vi "Error Clusters and Error Handling.vi"() -> ()   [LabVIEW 2023]
uses:
  <vilib>/Utility/error.llb/DialogType.ctl
panel:
  out "source":string
  out "code":i32
  out "status":bool
  out "Text from File":string
  in  "File Path":path=path "C:/Users/Barron Stone/Desktop/Exercise Files/CH06/06_04/begin/digits.txt"
  # "NOTE: Use the browse button to select the file path\nto \"digits.txt\" on your own computer."
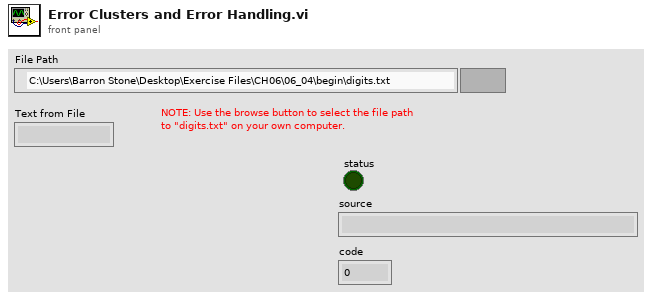
[diagram p1: front panel]
types:
  T1 = typedef "DialogType.ctl" = u16
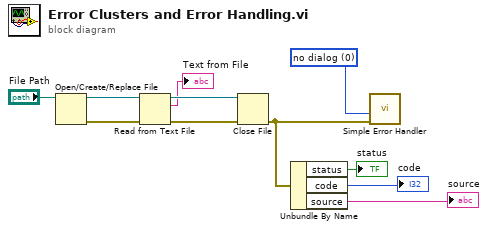
[diagram p0: block diagram]
diagram:
  w1 = T1 0 items=["no dialog", "OK message", "continue or stop message", "OK message + warnings", "continue/stop + warnings"] ("type of dialog (OK msg:1)")
  n1 = Open/Create/Replace File(file path (use dialog)="File Path") -> (refnum out=w10:refnum<file>, error out=w7:errorcluster)  [unwired: 5 in, 1 out]
  n2 = Read from Text File(file (use dialog)=w10, error in=w7) -> (refnum out=w9:refnum<file>, text=→"Text from File":string, error out=w6:errorcluster)  [unwired: 2 in, 1 out]
  n3 = Close File(refnum=w9, error in=w6) -> (error out=w2:errorcluster)  [unwired: 1 out]
  n4 = Unbundle By Name(w2) -> ("status"=→"status":bool, "code"=→"code":i32, "source"=→"source":string)
  n5 = call <vilib>:"Simple Error Handler.vi"("type of dialog (OK msg:1)"=w1, "error in (no error)"=w2) -> ()  [unwired: 3 in, 5 out]
